vi "FiberSpectrograph_getEvent_logLevel.vi"(8 "error in (no error)":errorcluster, 11 "logevent_logLevel_Ctl":T1) -> (0 "error out":errorcluster, 2 "function return":i32, 3 "logevent_logLevel_Ctl out":T1)   [LabVIEW 2016, in "SALLV_FiberSpectrograph.lvlib"]
doc: "int FiberSpectrograph_shm_getEvent_logLevelLV(FiberSpectrograph_logevent_logLevelLV *logevent_logLevel_Ctl );"
uses:
  SALLV_FiberSpectrograph.lvlib
  DataTypes/logevent_logLevel.ctl
  SALLV_FiberSpectrograph.so
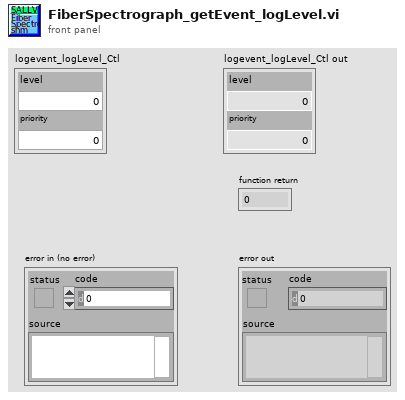
[diagram p1: front panel]
types:
  T1 = typedef "SALLV_FiberSpectrograph.lvlib/logevent_logLevel.ctl" = cluster{"level":i32, "priority":i32}
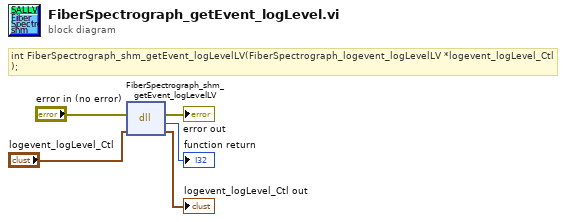
[diagram p0: block diagram]
diagram:
  # "int FiberSpectrograph_shm_getEvent_logLevelLV(FiberSpectrograph_logevent_logLevelLV *logevent_logLevel_Ctl );"
  n1 = dll-call lib="home/harini/SALLV_FiberSpectrograph/SALLV_FiberSpectrograph.*" fn="FiberSpectrograph_shm_getEvent_logLevelLV"(error in="error in (no error)", "logevent_logLevel_Ctl"="logevent_logLevel_Ctl") -> (error out=→"error out":errorcluster, →"function return":i32, "logevent_logLevel_Ctl"=→"logevent_logLevel_Ctl out":T1)  [unwired: 2 in, 1 out]
